vi "Detect Threshold.vi"(4 "error in (no error)":errorcluster, 5 "Amplitude":dbl, 7 "Action":T1) -> (0 "error out":errorcluster, 2 "Threshold":dbl)   [LabVIEW 2020]
doc: "The Detect Threshold VI modifies the current value of the threshold based on different events that occur during execution. Use <b>Action</b> to send commands:\n\n<b>Get Threshold</b> to return the current value of the threshold\n<b>Pulse Found</b> which sets the threshold close to the peak that was found\n<b>Pulse Not Found</b> which reduces the threshold to make peaks easier to find"
uses:
  Controls/Detect Threshold Control.ctl
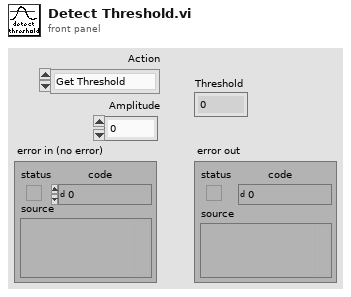
[diagram p1: front panel]
types:
  T1 = typedef "Detect Threshold Control.ctl" = enum16{"Get Threshold", "Pulse Found", "Pulse Not Found"}
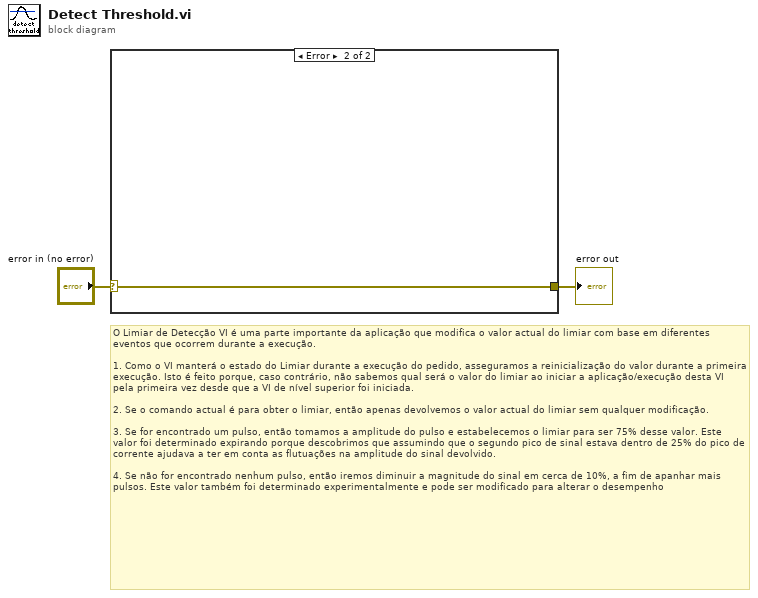
[diagram p0: block diagram]
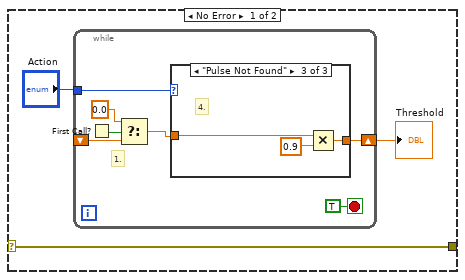
[diagram p2: hidden frame]
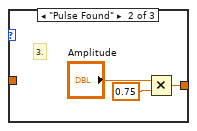
[diagram p4: hidden frame]
diagram:
  # "O Limiar de Detecção VI é uma parte importante da aplicação que modifica o valor actual do limiar com base em diferentes eventos que ocorrem durante a execução.\n\n1. Como o VI manterá o estado do Limiar durante a execução do pedido, asseguramos a reinicialização do valor durante a primeira execução. Isto é feito porque, caso contrário, não sabemos qual será o valor do limiar ao iniciar a aplicação/execução desta VI pela primeira vez desde que a VI de nível superior foi iniciada.\n\n2. Se o comando actual é para obter o limiar, então apenas devolvemos o valor actual do limiar sem qualquer modificação.\n\n3. Se for encontrado um pulso, então tomamos a amplitude do pulso e estabelecemos o limiar para ser 75% desse valor. Este valor foi determinado expirando porque descobrimos que assumindo que o segundo pico de sinal estava dentro de 25% do pico de corrente ajudava a ter em conta as flutuações na amplitude do sinal devolvido.\n\n4. Se não for encontrado nenhum pulso, então iremos diminuir a magnitude do sinal em cerca de 10%, a fim de apanhar mais pulsos. Este valor também foi determinado experimentalmente e pode ser modificado para alterar o desempenho"
  n1 = case shown="Error" "error in (no error)" {
    selector: "error in (no error)" -> [w5 w20]
    tunnel: [w5 w20] -> w1
    frame No Error {
      n2 = while {
        tunnel: "Action" -> [w12]
        shift-right: [w10] -> w4
        shift-left: _ -> [w8]
        stop <- TRUE stop-if-true
        # "1."
        n3 = First Call?() -> (First Call?: T/F=w9:bool)
        n4 = Select(t=0.0 ("element"), s=w9, f=w8) -> (s? t:f=w7:dbl)
        n5 = case shown="\"Pulse Not Found\"" w12 {
          tunnel: [w13 w14 w17] -> w10
          tunnel: w7 -> [w13 _ w18]
          frame "Get Threshold", Default {
            # "2."
          }
          frame "Pulse Found" {
            # "3."
            n6 = Multiply(x="Amplitude", y=0.75) -> (x*y=w14:dbl)
          }
          frame "Pulse Not Found" {
            # "4."
            n7 = Multiply(x=w18, y=0.9) -> (x*y=w17:dbl)
          }
        }
      }
      "Threshold" <- w4
    }
    frame Error {
    }
  }
  "error out" <- w1
